vi "5009 Subset Rectangles Not Equal.vi"(8 "error in (no error)":errorcluster) -> (0 "error out":errorcluster)   [LabVIEW 2020, in "MacroAssert.lvlib" / "Custom Errors.lvlib"]
uses:
  Custom Errors.lvlib
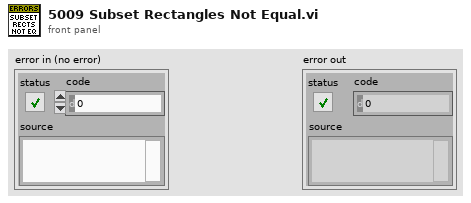
[diagram p1: front panel]
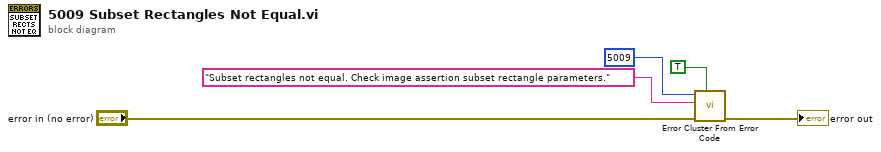
[diagram p0: block diagram]
diagram:
  n1 = call <vilib>:"Error Cluster From Error Code.vi"("show call chain? (False)"=TRUE, "error in (no error)"="error in (no error)", "error message (\"\")"="Subset rectangles not equal. Check image assertion subset rectangle parameters.", "error code (0)"=5009) -> ("error out"=→"error out":errorcluster)  [unwired: 5 in]
